vi "XML ( Get Node Value Single Input ).vi"(8 "error in (no error)":errorcluster, 10 "XPath expression":string, 11 "XML in":refnum<class "XML.lvclass">) -> (0 "error out":errorcluster, 2 "Value":string, 3 "XML out":refnum<class "XML.lvclass">)   [LabVIEW 2018, in "XML.lvlib" / "XML.lvclass"]
uses:
  XML.lvclass
  XML.lvclass/XML.ctl
  <vilib>/xml/Close Reference(Node).vi
  <vilib>/xml/NI_XML.lvlib
  <resource>/objmgr/DOMUserDefRef.rc
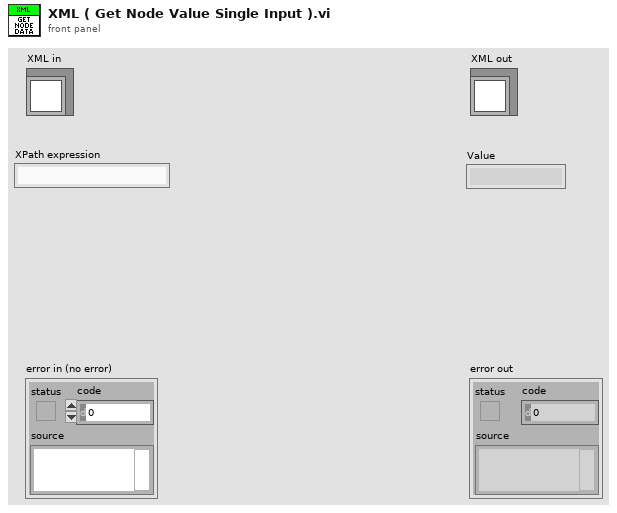
[diagram p1: front panel]
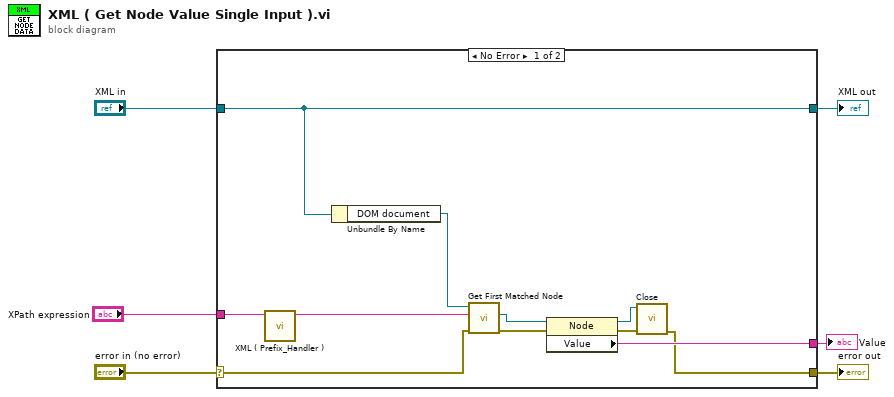
[diagram p0: block diagram]
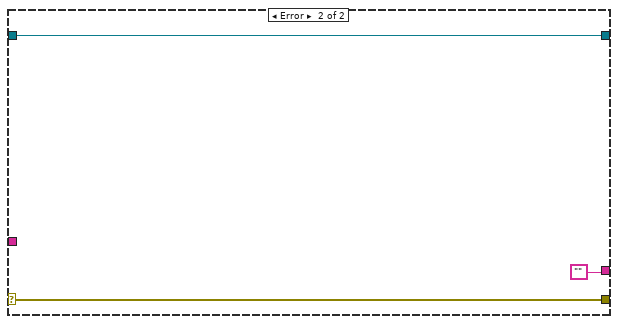
[diagram p2: hidden frame]
diagram:
  n1 = case shown="No Error" "error in (no error)" {
    selector: "error in (no error)" -> [w13 w20]
    tunnel: [w9 w20] -> w5
    tunnel: [w17 w19] -> w3
    tunnel: "XML in" -> [w17 w19]
    tunnel: [w10 ""] -> w2
    tunnel: "XPath expression" -> [w8 _]
    frame No Error {
      n2 = call "XML ( Prefix_Handler ).vi"("input string"=w8) -> ("result string"=w7:string)  [unwired: 10 in]
      n3 = Unbundle By Name(w17) -> ("DOM document"=w14:refnum<k20>)
      n4 = call <vilib>:"Get First Matched Node.vi"("error in (no error)"=w13, "XPath expression"=w7, "node in"=w14) -> ("error out"=w15:errorcluster, "node result"=w16:refnum<k20>)  [unwired: 6 in, 1 out]
      n5 = property class="Node"(reference=w16, error in=w15) -> (reference out=w11:refnum<k20>, error out=w12:errorcluster, "Value"=w10:string)
      n6 = call-poly <vilib>:"Close.vi"("error in (no error)"=w12, "node"=w11) -> ("error out"=w9:errorcluster)  [unwired: 7 in]
    }
    frame Error {
    }
  }
  "error out" <- w5
  "XML out" <- w3
  "Value" <- w2
